vi "Sine Wave Chart (While Loop with Runtime Options).vi"() -> ()   [LabVIEW 2017]
panel:
  in  "Enum":enum16{"Black", "Red", "Green", "Blue"}(ring)
  in  "Clear Chart?":bool
  out "Waveform Chart":dbl(graph)
  in  "stop":bool
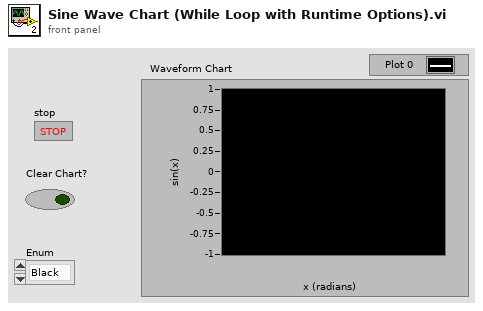
[diagram p1: front panel]
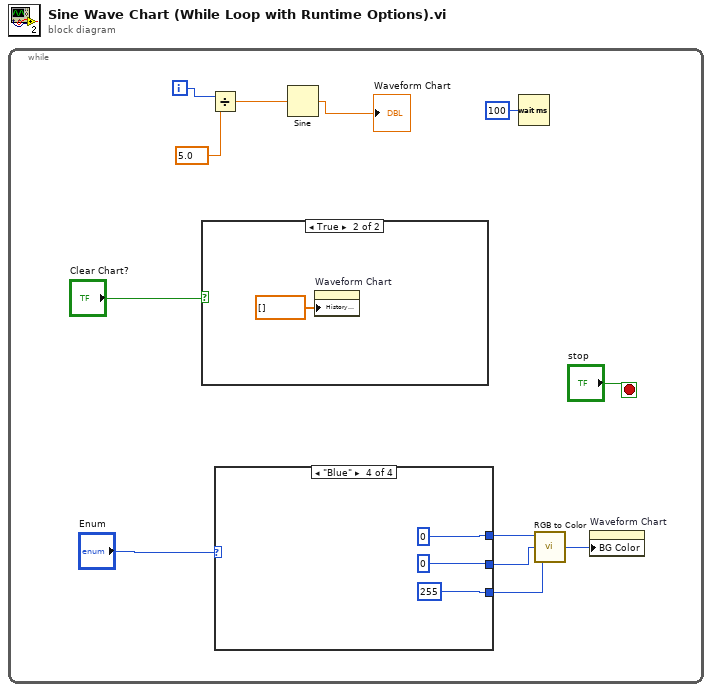
[diagram p0: block diagram]
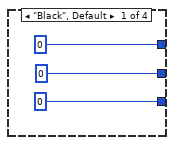
[diagram p2: hidden frame]
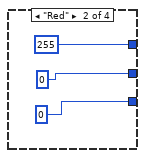
[diagram p3: hidden frame]
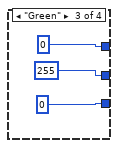
[diagram p4: hidden frame]
diagram:
  n1 = while {
    i -> [w10]
    stop <- "stop" stop-if-true
    n2 = case shown="True" "Clear Chart?" {
      frame False {
      }
      frame True {
        n3 = property on="Waveform Chart" class="WFChart (strict)"("History Data"=dbl[] []) -> ()  [unwired: 2 in, 2 out]
      }
    }
    n4 = Divide(x=w10, y=5.0) -> (x/y=w8:dbl)
    n5 = case shown="\"Blue\"" "Enum" {
      tunnel: [u8 0 u8 255 u8 0 u8 0] -> w3
      tunnel: [u8 0 u8 0 u8 255 u8 0] -> w2
      tunnel: [u8 0 u8 0 u8 0 u8 255] -> w1
      frame "Black", Default {
      }
      frame "Red" {
      }
      frame "Green" {
      }
      frame "Blue" {
      }
    }
    n6 = Sine(x=w8) -> (sin(x)=→"Waveform Chart":dbl)
    n7 = Wait (ms)(milliseconds to wait=u32 100) -> ()  [unwired: 1 out]
    n8 = call <vilib>:"RGB to Color.vi"("B"=w1, "G"=w2, "R"=w3) -> ("Color"=w4:u32)
    n9 = property on="Waveform Chart" class="WFChart (strict)"("BG Color"=w4) -> ()  [unwired: 2 in, 2 out]
  }
